vi "setTrigger6009.vi"(8 "error in (no error)":errorcluster, 9 "Device Name in":string, 10 "Trigger":bool, 11 "Refnum in":refnum<k21>) -> (0 "error out":errorcluster, 1 "Device Name out":string, 3 "Refnum out":refnum<k21>)   [LabVIEW 2011]
uses:
  C:/Program Files/National Instruments/LabVIEW 2011/resource/objmgr/daqmx.rc
panel:
  out "NumChans":u32
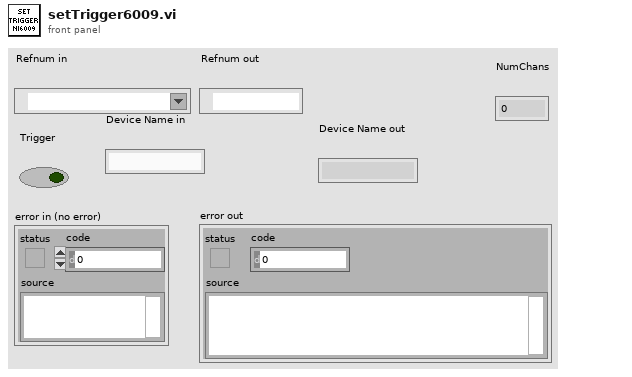
[diagram p1: front panel]
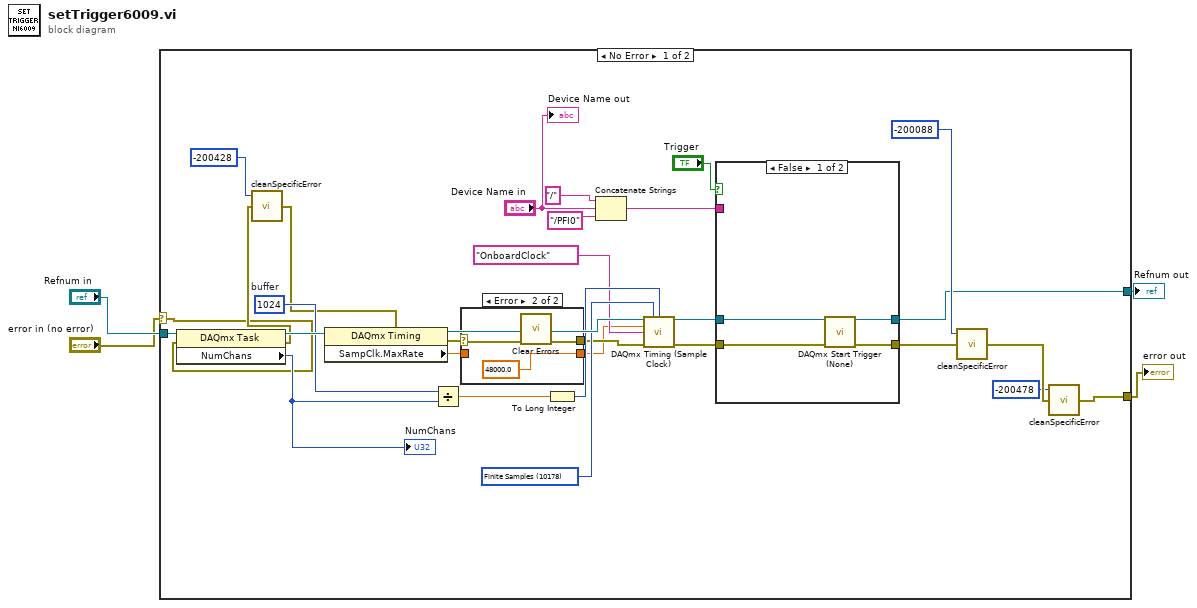
[diagram p0: block diagram]
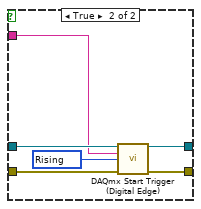
[diagram p3: hidden frame]
diagram:
  n1 = case shown="No Error" "error in (no error)" {
    selector: "error in (no error)" -> [w5 w50]
    tunnel: [w29 w51] -> w4
    tunnel: "Refnum in" -> [w11 w51]
    tunnel: [w6 w50] -> w2
    frame No Error {
      w22 = 10178 items=["Finite Samples"=10178, "Continuous Samples"=10123, "Hardware Timed Single Point"=12522] ("sample mode")
      w25 = 1024  # buffer
      n2 = property class="DAQmx Task"(reference=w11, error in=w5) -> (reference out=w28:refnum<k21>, error out=w15:errorcluster, "NumChans"=w26:u32)
      "NumChans" <- w26
      n3 = call "cleanSpecificError.vi"("error out"=w15, "error code"=-200428) -> ("error IO"=w14:errorcluster)  [unwired: 2 in, 1 out]
      n4 = property class="DAQmx Timing"(reference=w28, error in=w14) -> (reference out=w27:refnum<k21>, error out=w10:errorcluster, "SampClk.MaxRate"=w8:dbl)
      n5 = Divide(x=w25, y=w26) -> (x/y=w24:dbl)
      n6 = case shown="Error" w10 {
        selector: w10 -> [w36 w37]
        tunnel: [w36 w38] -> w9
        tunnel: w8 -> [w35 _]
        tunnel: [w35 48000.0] -> w7
        frame No Error {
        }
        frame Error {
          n7 = call "Clear Errors.vi"("error in (no error)"=w37) -> ("error out"=w38:errorcluster)  [unwired: 6 in]
        }
      }
      n8 = To Long Integer(number=w24) -> (32bit integer=w23:i32)
      n9 = Concatenate Strings("/" ("string"), "Device Name in", "/PFI0") -> (w17:string)
      n10 = call "DAQmx Timing (Sample Clock).vi"("task/channels in"=w27, "sample mode"=w22, "samples per channel"=w23, "rate"=w7, "source"=tag "OnboardClock", "error in"=w9) -> ("task out"=w34:refnum<k21>, "error out"=w33:errorcluster)  [unwired: 8 in]
      n11 = case shown="False" "Trigger" {
        tunnel: w34 -> [w41 w49]
        tunnel: [w43 w48] -> w29
        tunnel: w33 -> [w40 w46]
        tunnel: [w42 w45] -> w30
        tunnel: w17 -> [_ w44]
        frame False {
          n12 = call "DAQmx Start Trigger (None).vi"("task/channels in"=w41, "error in"=w40) -> ("task out"=w43:refnum<k21>, "error out"=w42:errorcluster)  [unwired: 12 in]
        }
        frame True {
          w47 = 10280 items=["Rising"=10280, "Falling"=10171] ("edge")
          n13 = call "DAQmx Start Trigger (Digital Edge).vi"("task/channels in"=w49, "source"=w44, "edge"=w47, "error in"=w46) -> ("task out"=w48:refnum<k21>, "error out"=w45:errorcluster)  [unwired: 10 in]
        }
      }
      n14 = call "cleanSpecificError.vi"("error out"=w30, "error code"=-200088) -> ("error IO"=w13:errorcluster)  [unwired: 2 in, 1 out]
      n15 = call "cleanSpecificError.vi"("error out"=w13, "error code"=-200478) -> ("error IO"=w6:errorcluster)  [unwired: 2 in, 1 out]
      "Device Name out" <- "Device Name in"
    }
    frame Error {
    }
  }
  "Refnum out" <- w4
  "error out" <- w2
